vi "ClearFaults.vi"(11 "Sig_AI in":refnum<class "AI.lvclass">) -> (3 "Sig_AI out":refnum<class "AI.lvclass">)   [LabVIEW 2019, in "AI.lvclass"]
uses:
  AI.lvclass
  AI.lvclass/AI.ctl
  AnalogComparator_class/AnalogComparator.lvclass
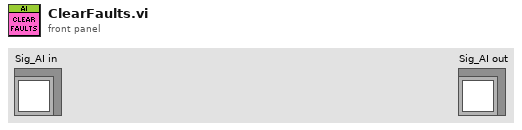
[diagram p1: front panel]
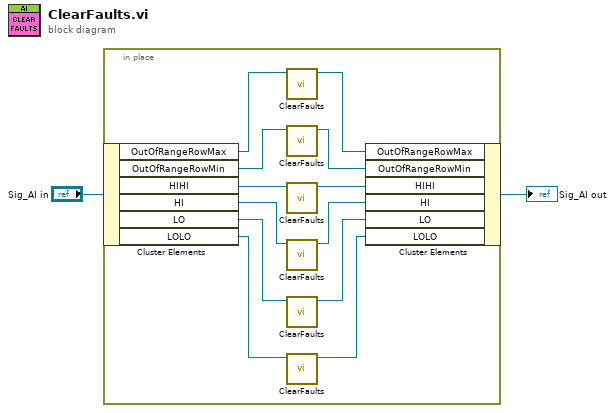
[diagram p0: block diagram]
diagram:
  n1 = in-place {
    n2 = in-place-cluster #1("Sig_AI in") -> ("OutOfRangeRowMax"=w14:refnum<class "AnalogComparator.lvclass">, "OutOfRangeRowMin"=w12:refnum<class "AnalogComparator.lvclass">, "HIHI"=w11:refnum<class "AnalogComparator.lvclass">, "HI"=w10:refnum<class "AnalogComparator.lvclass">, "LO"=w9:refnum<class "AnalogComparator.lvclass">, "LOLO"=w8:refnum<class "AnalogComparator.lvclass">)
    n3 = call-dynamic "ClearFaults.vi"("class data in"=w14) -> ("class data out"=w13:refnum<class "AnalogComparator.lvclass">)  [unwired: 10 in]
    n4 = call-dynamic "ClearFaults.vi"("class data in"=w12) -> ("class data out"=w7:refnum<class "AnalogComparator.lvclass">)  [unwired: 10 in]
    n5 = call-dynamic "ClearFaults.vi"("class data in"=w11) -> ("class data out"=w6:refnum<class "AnalogComparator.lvclass">)  [unwired: 10 in]
    n6 = call-dynamic "ClearFaults.vi"("class data in"=w10) -> ("class data out"=w5:refnum<class "AnalogComparator.lvclass">)  [unwired: 10 in]
    n7 = call-dynamic "ClearFaults.vi"("class data in"=w9) -> ("class data out"=w4:refnum<class "AnalogComparator.lvclass">)  [unwired: 10 in]
    n8 = call-dynamic "ClearFaults.vi"("class data in"=w8) -> ("class data out"=w3:refnum<class "AnalogComparator.lvclass">)  [unwired: 10 in]
    n9 = in-place-cluster #1("OutOfRangeRowMax"=w13, "OutOfRangeRowMin"=w7, "HIHI"=w6, "HI"=w5, "LO"=w4, "LOLO"=w3) -> (→"Sig_AI out":refnum<class "AI.lvclass">)
  }
